vi "MicronsToSetting.vi"(9 "Scan Settings":T1={"XStart"=-200000000, "XEnd"=200000000, "XNum"=500, "YStart"=-200000000, "YEnd"=200000000, "YNum"=500, "ZStart"=0, "ZEnd"=0, "ZNum"=1}, 10 "Scan Settings (um)":T1={"XStart"=-100, "XEnd"=100, "XNum"=250, "YStart"=-100, "YEnd"=100, "YNum"=250, "ZStart"=-50, "ZEnd"=50, "ZNum"=30}, 11 "Microns (X,Y,Z)":dbl[](array[numeric])) -> (3 "Setting":i32[](array[numeric]))   [LabVIEW 2014]
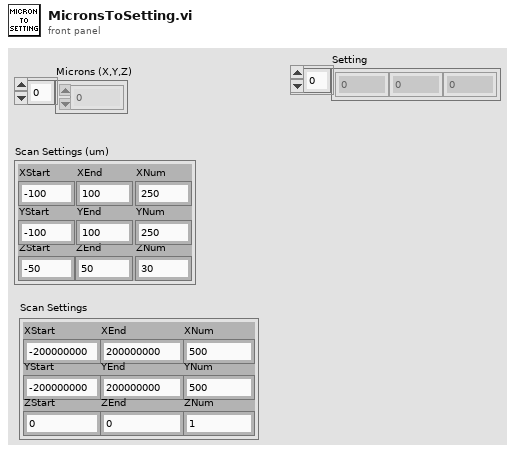
[diagram p1: front panel]
types:
  T1 = cluster{"XStart":i32, "XEnd":i32, "XNum":i32, "YStart":i32, "YEnd":i32, "YNum":i32, "ZStart":i32, "ZEnd":i32, "ZNum":i32}
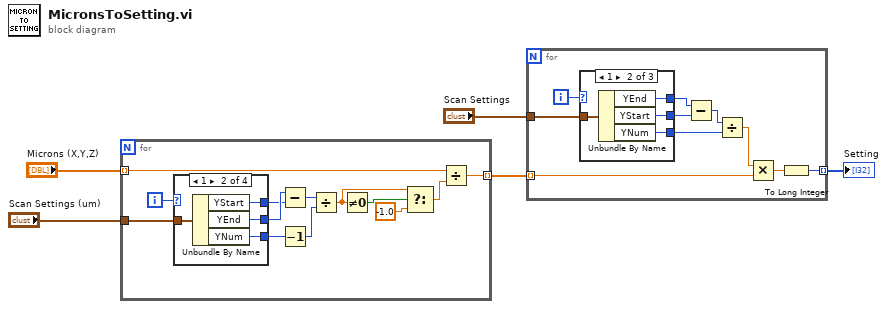
[diagram p0: block diagram]
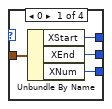
[diagram p2: hidden frame]
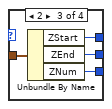
[diagram p3: hidden frame]
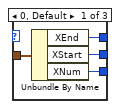
[diagram p5: hidden frame]
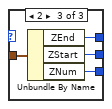
[diagram p6: hidden frame]
diagram:
  n1 = for {
    tunnel: "Scan Settings (um)" -> [w17]
    tunnel: "Microns (X,Y,Z)" -> [w6] mode=indexing
    tunnel: [w8] -> w1 mode=indexing
    i -> [w18]
    n2 = case shown="1" w18 {
      tunnel: w17 -> [w20 w24 w30 _]
      tunnel: [w21 w25 w29 _] -> w16
      tunnel: [w22 w26 w28 _] -> w7
      tunnel: [w19 w23 w27 _] -> w14
      frame 0 {
        n3 = Unbundle By Name(w20) -> ("XStart"=w22:i32, "XEnd"=w21:i32, "XNum"=w19:i32)
      }
      frame 1 {
        n4 = Unbundle By Name(w24) -> ("YStart"=w26:i32, "YEnd"=w25:i32, "YNum"=w23:i32)
      }
      frame 2 {
        n5 = Unbundle By Name(w30) -> ("ZStart"=w28:i32, "ZEnd"=w29:i32, "ZNum"=w27:i32)
      }
      frame Default {
      }
    }
    n6 = Subtract(x=w16, y=w7) -> (x-y=w15:i32)
    n7 = Decrement(x=w14) -> (x-1=w13:i32)
    n8 = Divide(x=w15, y=w13) -> (x/y=w11:dbl)
    n9 = Not Equal To 0?(x=w11) -> (x != 0?=w12:bool)
    n10 = Select(t=w11, s=w12, f=-1.0) -> (s? t:f=w10:dbl)
    n11 = Divide(x=w6, y=w10) -> (x/y=w8:dbl)
  }
  n12 = for {
    tunnel: w1 -> [w35] mode=indexing
    tunnel: "Scan Settings" -> [w40]
    tunnel: [w33] -> w4 mode=indexing
    i -> [w39]
    n13 = case shown="1" w39 {
      tunnel: w40 -> [w44 w48 w52]
      tunnel: [w43 w47 w51] -> w36
      tunnel: [w42 w46 w50] -> w34
      tunnel: [w41 w45 w49] -> w37
      frame 0, Default {
        n14 = Unbundle By Name(w44) -> ("XEnd"=w43:i32, "XStart"=w42:i32, "XNum"=w41:i32)
      }
      frame 1 {
        n15 = Unbundle By Name(w48) -> ("YEnd"=w47:i32, "YStart"=w46:i32, "YNum"=w45:i32)
      }
      frame 2 {
        n16 = Unbundle By Name(w52) -> ("ZEnd"=w51:i32, "ZStart"=w50:i32, "ZNum"=w49:i32)
      }
    }
    n17 = Subtract(x=w36, y=w34) -> (x-y=w38:i32)
    n18 = Divide(x=w38, y=w37) -> (x/y=w32:dbl)
    n19 = Multiply(x=w32, y=w35) -> (x*y=w31:dbl)
    n20 = To Long Integer(number=w31) -> (32bit integer=w33:i32)
  }
  "Setting" <- w4
